vi "IMAQ Initialize.vi"(8 "error in":errorcluster) -> (0 "error out":errorcluster, 3 "Multiple Image Cluster":T2)   [LabVIEW 2020]
uses:
  <vilib>/vision/Image Controls.llb/IMAQ Image.ctl
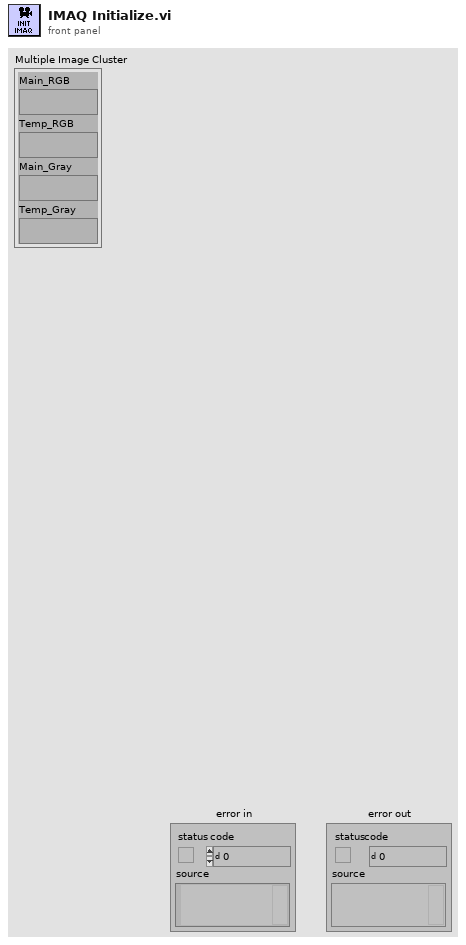
[diagram p1: front panel]
types:
  T1 = typedef "IMAQ Image.ctl" = refnum<image>
  T2 = cluster{"Main_RGB":T1, "Temp_RGB":T1, "Main_Gray":T1, "Temp_Gray":T1}
  T3 = typedef "Image Type" = u32
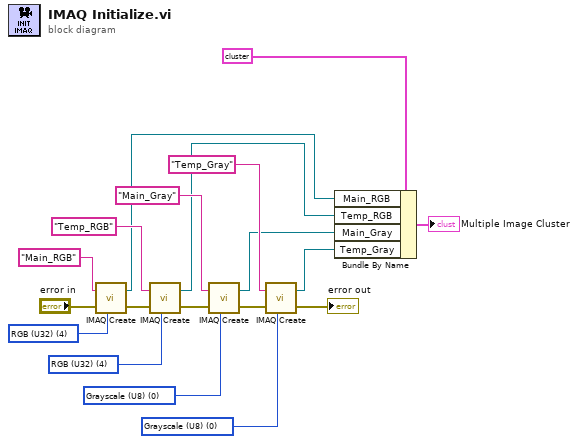
[diagram p0: block diagram]
diagram:
  w15 = T3 4 items=["Grayscale (U8)", "Grayscale (I16)", "Grayscale (SGL)", "Complex (CSG)", "RGB (U32)", "HSL (U32)", "RGB (U64)", "Grayscale (U16)"] ("Image Type")
  w16 = T3 4 items=["Grayscale (U8)", "Grayscale (I16)", "Grayscale (SGL)", "Complex (CSG)", "RGB (U32)", "HSL (U32)", "RGB (U64)", "Grayscale (U16)"] ("Image Type")
  w18 = T3 0 items=["Grayscale (U8)", "Grayscale (I16)", "Grayscale (SGL)", "Complex (CSG)", "RGB (U32)", "HSL (U32)", "RGB (U64)", "Grayscale (U16)"] ("Image Type")
  w17 = T3 0 items=["Grayscale (U8)", "Grayscale (I16)", "Grayscale (SGL)", "Complex (CSG)", "RGB (U32)", "HSL (U32)", "RGB (U64)", "Grayscale (U16)"] ("Image Type")
  n1 = call "IMAQ Create"("Image Name"="Main_RGB", "Image Type"=w16, "error in (no error)"="error in") -> ("New Image"=w7:T1, "error out"=w14:errorcluster)  [unwired: 2 in]
  n2 = call "IMAQ Create"("Image Name"="Temp_RGB", "Image Type"=w15, "error in (no error)"=w14) -> ("New Image"=w6:T1, "error out"=w13:errorcluster)  [unwired: 2 in]
  n3 = call "IMAQ Create"("Image Name"="Main_Gray", "Image Type"=w17, "error in (no error)"=w13) -> ("New Image"=w5:T1, "error out"=w19:errorcluster)  [unwired: 2 in]
  n4 = call "IMAQ Create"("Image Name"="Temp_Gray", "Image Type"=w18, "error in (no error)"=w19) -> ("New Image"=w4:T1, "error out"=→"error out":errorcluster)  [unwired: 2 in]
  n5 = Bundle By Name(cluster=T2 {"Main_RGB"=refnum, "Temp_RGB"=refnum, "Main_Gray"=refnum, "Temp_Gray"=refnum} ("Capture Image"), "Main_RGB"=w7, "Temp_RGB"=w6, "Main_Gray"=w5, "Temp_Gray"=w4) -> (→"Multiple Image Cluster":T2)
